vi "_nPoints Concept - Hall Effect.vi"() -> ()   [LabVIEW 2013]
uses:
  <vilib>/DAQmx/create/channels.llb/DAQmx Create Channel (AI-Voltage-Basic).vi
  <vilib>/DAQmx/read.llb/DAQmx Read (Analog DBL 1Chan 1Samp).vi
panel:
  out "Meter":dbl(knob) scale=0.0..5.0
  in  "Gravity":dbl(slide)=0.0059880239520958695 scale=-1.0..1.0
  in  "X Max":i32=410
  out "Array":cluster{"X":i32, "Y":i32}[](array[cluster])
  in  "px/s":i32=250
  in  "Seperation":i32=40
  in  "Origin":cluster{"X":i32, "Y":i32}={"X"=300, "Y"=150}
  out "new picture 2":picture
  in  "Jitter":dbl=1.0
  in  "Number of Particles":u32=10
  in  "milliseconds to wait":u32=50
  out "Waveform Chart":dbl(graph)
  in  "Stop Button":bool
  # "Hall Effect Sensor"
  # "+5V"
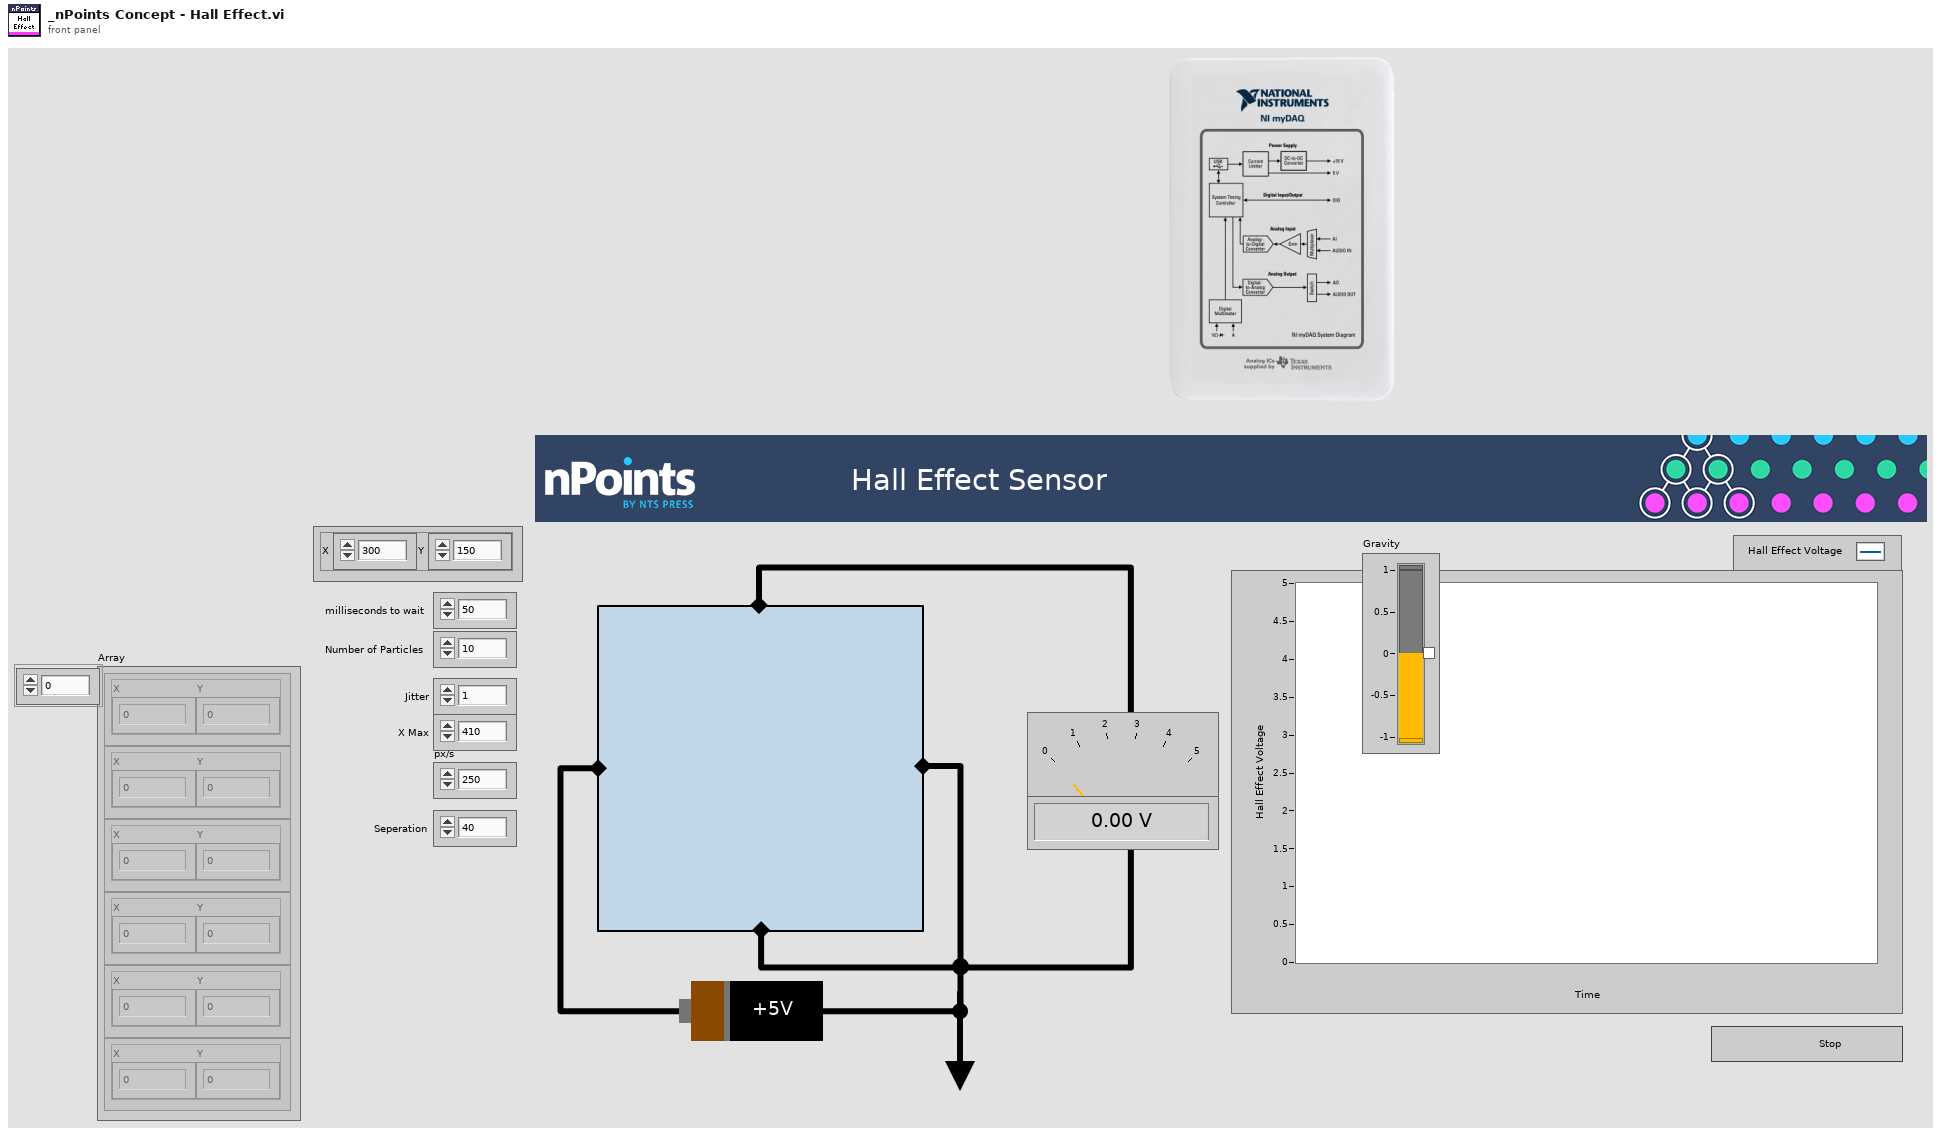
[diagram p1: front panel]
types:
  T1 = typedef "imagedata.ctl" = cluster{"image type":i32, "image depth":i32, "image":u8[], "mask":u8[], "colors":u32[], "Rectangle":cluster{"left":i16, "top":i16, "right":i16, "bottom":i16}}
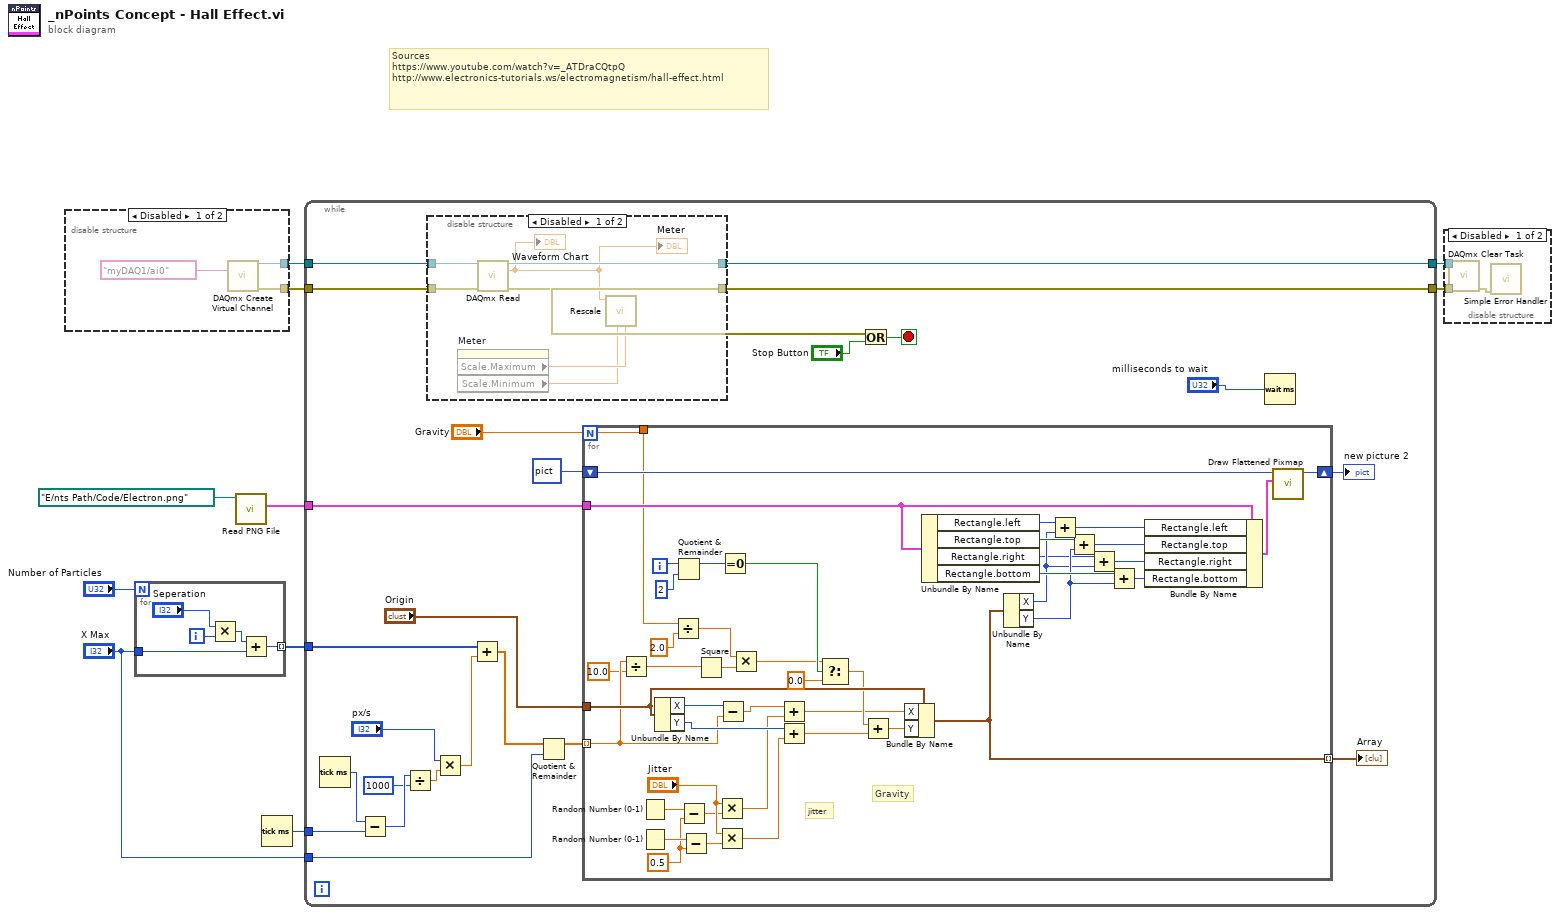
[diagram p0: block diagram]
diagram:
  # "Sources\nhttps://www.youtube.com/watch?v=_ATDraCQtpQ\nhttp://www.electronics-tutorials.ws/electromagnetism/hall-effect.html"
  n1 = disable-structure shown="Disabled" {
    disable-tunnel: [w12 _] -> w4
    disable-tunnel: [w11 _] -> w3
    frame Disabled {
      n2 = call-poly <vilib>:"DAQmx Create Virtual Channel.vi"("physical channels"=tag "myDAQ1/ai0") -> ("task out"=w12:refnum<k21>, "error out"=w11:errorcluster)  [unwired: 13 in]
    }
    frame Enabled {
    }
  }
  n3 = for {
    N: "Number of Particles" -> [_]
    tunnel: [w15] -> w8 mode=indexing
    tunnel: "X Max" -> [w14]
    i -> [w16]
    n4 = Multiply(x="Seperation", y=w16) -> (x*y=w17:i32)
    n5 = Add(x=w17, y=w14) -> (x+y=w15:i32)
  }
  n6 = call <vilib>:"Read PNG File.vi"("path to PNG file"=path "E:/nts Path/Code/Electron.png") -> ("image data"=w9:T1)  [unwired: 8 in, 2 out]
  n7 = Tick Count (ms)() -> (millisecond timer value=w7:u32)
  n8 = while {
    tunnel: w9 -> [w37]
    tunnel: w8 -> [w40]
    tunnel: w7 -> [w33]
    tunnel: "X Max" -> [w28]
    tunnel: w4 -> [w26]
    tunnel: w3 -> [w25]
    tunnel: [w24] -> w2
    tunnel: [w23] -> w1
    stop <- w22 stop-if-true
    n9 = Tick Count (ms)() -> (millisecond timer value=w35:u32)
    n10 = Subtract(x=w35, y=w33) -> (x-y=w34:u32)
    n11 = Divide(x=w34, y=u32 1000) -> (x/y=w31:dbl)
    n12 = disable-structure shown="Disabled" {
      disable-tunnel: w26 -> [w49 _]
      disable-tunnel: w25 -> [w48 _]
      disable-tunnel: [w47 _] -> w24
      disable-tunnel: [w46 _] -> w23
      frame Disabled {
        n13 = property on="Meter" class="Knob (strict)"() -> ("Scale.Maximum"=w44:dbl, "Scale.Minimum"=w43:dbl)  [unwired: 2 in, 2 out]
        n14 = call-poly <vilib>:"DAQmx Read.vi"("task/channels in"=w49, "error in"=w48) -> ("task out"=w46:refnum<k21>, "data"=w45:dbl, "error out"=w47:errorcluster)  [unwired: 11 in]
        "Waveform Chart" <- w45
        "Meter" <- w45
        n15 = call "Rescale.vi"("Max In"=w44, "Min In"=w43, "Input"=w45) -> ()  [unwired: 8 in, 1 out]
      }
      frame Enabled {
      }
    }
    n16 = Multiply(x="px/s", y=w31) -> (x*y=w29:dbl)
    n17 = Add(x=w40, y=w29) -> (x+y=w39:dbl[])
    n18 = Quotient & Remainder(x=w39, y=w28) -> (x-y*floor(x/y)=w27:dbl[])  [unwired: 1 out]
    n19 = for {
      shift-right: [w93] -> w42
      shift-left: picture data[5B] ("new picture") -> [w92]
      tunnel: w27 -> [w52] mode=indexing
      tunnel: "Origin" -> [w90]
      tunnel: w37 -> [w79]
      tunnel: [w77] -> w36 mode=indexing
      tunnel: "Gravity" -> [w50]
      i -> [w57]
      w73 = 0.5 ("Rand Scale")
      # "Gravity"
      # "jitter"
      n20 = Divide(x=w52, y=10.0 ("x")) -> (x/y=w53:dbl)
      n21 = Random Number (0-1)() -> (number: 0 to 1=w75:dbl)
      n22 = Random Number (0-1)() -> (number: 0 to 1=w74:dbl)
      n23 = Unbundle By Name(w90) -> ("X"=w91:i32, "Y"=w70:i32)
      n24 = Divide(x=w50, y=2.0 ("x")) -> (x/y=w56:dbl)
      n25 = Quotient & Remainder(x=w57, y=2) -> (x-y*floor(x/y)=w66:i32)  [unwired: 1 out]
      n26 = Subtract(x=w75, y=w73) -> (x-y=w72:dbl)
      n27 = Subtract(x=w74, y=w73) -> (x-y=w71:dbl)
      n28 = Square(x=w53) -> (x^2=w54:dbl)
      n29 = Multiply(x="Jitter", y=w72) -> (x*y=w69:dbl)
      n30 = Multiply(x="Jitter", y=w71) -> (x*y=w68:dbl)
      n31 = Subtract(x=w91, y=w52) -> (x-y=w65:dbl)
      n32 = Equal To 0?(x=w66) -> (x = 0?=w64:bool)
      n33 = Multiply(x=w56, y=w54) -> (x*y=w63:dbl)
      n34 = Add(x=w65, y=w69) -> (x+y=w60:dbl)
      n35 = Add(x=w70, y=w68) -> (x+y=w59:dbl)
      n36 = Select(t=w63, s=w64, f=0.0) -> (s? t:f=w61:dbl)
      n37 = Add(x=w61, y=w59) -> (x+y=w58:dbl)
      n38 = Bundle By Name(cluster=w90, "X"=w60, "Y"=w58) -> (w77:cluster{"X":i32, "Y":i32})
      n39 = Unbundle By Name(w79) -> ("Rectangle.left"=w80:i16, "Rectangle.top"=w86:i16, "Rectangle.right"=w82:i16, "Rectangle.bottom"=w88:i16)
      n40 = Unbundle By Name(w77) -> ("X"=w83:i32, "Y"=w85:i32)
      n41 = Add(x=w80, y=w83) -> (x+y=w81:i32)
      n42 = Add(x=w86, y=w85) -> (x+y=w87:i32)
      n43 = Add(x=w82, y=w83) -> (x+y=w84:i32)
      n44 = Add(x=w88, y=w85) -> (x+y=w89:i32)
      n45 = Bundle By Name(cluster=w79, "Rectangle.left"=w81, "Rectangle.top"=w87, "Rectangle.right"=w84, "Rectangle.bottom"=w89) -> (w78:T1)
      n46 = call <vilib>:"Draw Flattened Pixmap.vi"("image data"=w78, "picture"=w92) -> ("new picture"=w93:picture)  [unwired: 7 in]
    }
    "new picture 2" <- w42
    "Array" <- w36
    n47 = Or(x=w24, y="Stop Button") -> (x .or. y?=w22:bool)
    n48 = Wait (ms)(milliseconds to wait="milliseconds to wait") -> ()  [unwired: 1 out]
  }
  n49 = disable-structure shown="Disabled" {
    disable-tunnel: w2 -> [w95 _]
    disable-tunnel: w1 -> [w94 _]
    frame Disabled {
      n50 = call <vilib>:"DAQmx Clear Task.vi"("task in"=w94, "error in"=w95) -> ("error out"=w96:errorcluster)  [unwired: 13 in]
      n51 = call <vilib>:"Simple Error Handler.vi"("error in (no error)"=w96) -> ()  [unwired: 4 in, 5 out]
    }
    frame Enabled {
    }
  }
